vi "Generation word specific.vi"(0 "Template Path":path, 1 "paper size (letter)":i32(ring)=2 items=["wdPaper10x14", "wdPaper11x17", "wdPaperLetter", "wdPaperLetterSmall", "wdPaperLegal", "wdPaperExecutive", "wdPaperA3", "wdPaperA4", "wdPaperA4Small", "wdPaperA5", "wdPaperB4", "wdPaperB5", "wdPaperCSheet", "wdPaperDSheet", "wdPaperESheet", "wdPaperFanfoldLegalGerman", "wdPaperFanfoldStdGerman", "wdPaperFanfoldUS", "wdPaperFolio", "wdPaperLedger", "wdPaperNote", "wdPaperQuarto", "wdPaperStatement", "wdPaperTabloid", "wdPaperEnvelope9", "wdPaperEnvelope10", "wdPaperEnvelope11", "wdPaperEnvelope12", "wdPaperEnvelope14", "wdPaperEnvelopeB4", "wdPaperEnvelopeB5", "wdPaperEnvelopeB6", "wdPaperEnvelopeC3", "wdPaperEnvelopeC4", "wdPaperEnvelopeC5", "wdPaperEnvelopeC6", "wdPaperEnvelopeC65", "wdPaperEnvelopeDL", "wdPaperEnvelopeItaly", "wdPaperEnvelopeMonarch", "wdPaperEnvelopePersonal", "wdPaperCustom"], 2 "Data Set Name":string, 3 "column headers":string[](array[string]), 4 "Table Data":string[][](array[string]), 5 "error in (no error)":errorcluster) -> (14 "Report Saved Path":path, 19 "error out":errorcluster)   [LabVIEW 2020]
uses:
  <vilib>/Utility/NIReport.llb/Report Type.ctl
  <vilib>/addons/_office/_exclsub.llb/font.ctl
  <vilib>/Utility/NIReport.llb/Append Text Table to Report (wrap).vi
  <vilib>/addons/_office/word.llb/Word Edit Cell ([str]).vi
  <vilib>/Utility/NIReport.llb/NI_report.lvclass
  <vilib>/Utility/NIReport.llb/NI_ReportGenerationCore.lvlib
  <vilib>/Utility/NIReport.llb/Word/NI_Word.lvclass
  <vilib>/addons/_office/NI_ReportGenerationToolkit.lvlib
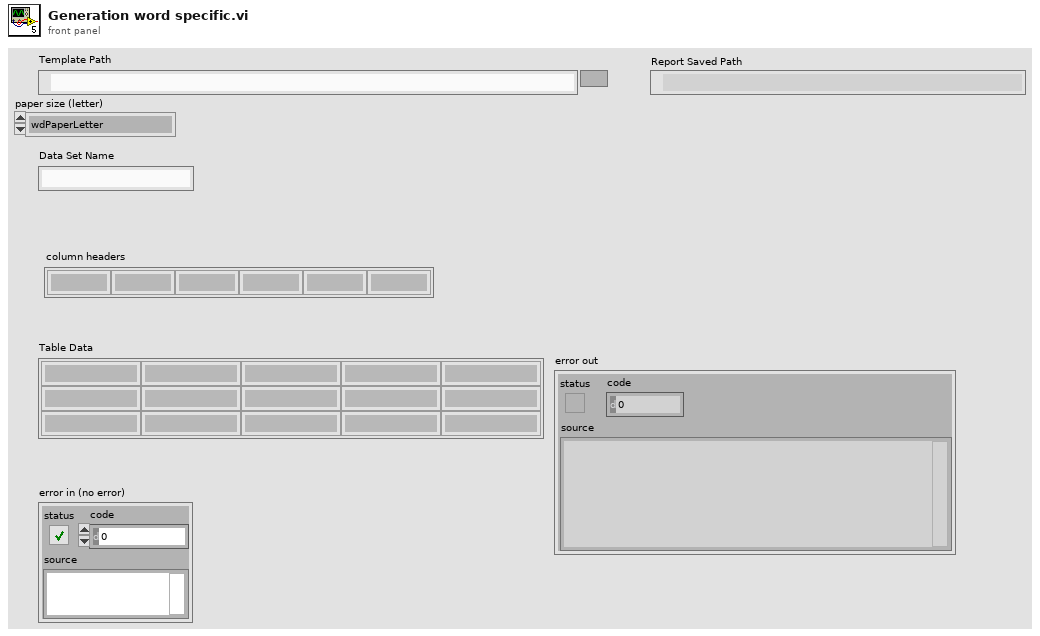
[diagram p1: front panel]
types:
  T1 = typedef "NI_ReportGenerationToolkit.lvlib/font.ctl" = cluster{"font name":string, "font size":dbl, "bold":u16, "italic":u16, "underline":u16, "strike through":u16, "font color":u32}
  T2 = typedef "NI_ReportGenerationCore.lvlib/Report Type.ctl" = enum16{"HTML", "Word", "Excel"}
  T3 = enum16{"maximized", "minimized", "normal", "no change"}
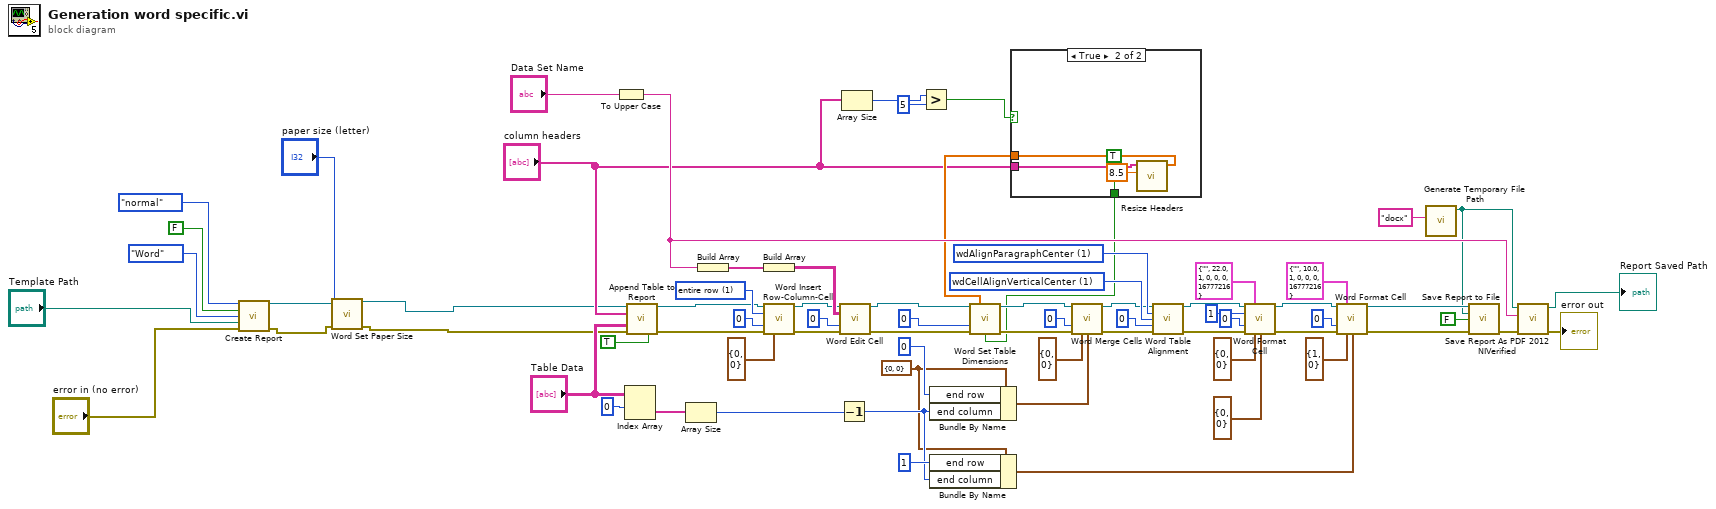
[diagram p0: block diagram]
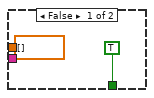
[diagram p2: hidden frame]
diagram:
  w54 = u16 1 items=["shift cells right", "entire row", "entire column"] ("mode (entire column)")
  w24 = cluster{"end row":i32, "end column":i32} {"end row"=0, "end column"=0} ("end")
  w64 = 1 items=["wdCellAlignVerticalTop"=0, "wdCellAlignVerticalCenter"=1, "wdCellAlignVerticalBottom"=3] ("vertical alignment (top)")
  w65 = 1 items=["wdAlignParagraphLeft"=0, "wdAlignParagraphCenter"=1, "wdAlignParagraphRight"=2, "wdAlignParagraphJustify"=3, "wdAlignParagraphDistribute"=4, "wdAlignParagraphJustifyMed"=5, "wdAlignParagraphJustifyHi"=7, "wdAlignParagraphJustifyLow"=8] ("horizontal alignment (left)")
  n1 = call <vilib>:"Create Report.vi"("window state (normal)"=T3."normal", "display alerts? (F)"=FALSE, "report type"=Report_Type."Word", "template (empty)"="Template Path", "error in (no error)"="error in (no error)") -> ("report out"=w6:refnum<class "NI_report.lvclass">, "error out"=w3:errorcluster)  [unwired: 9 in]
  n2 = call <vilib>:"Word Set Paper Size.vi"("report in"=w6, "paper size (letter)"="paper size (letter)", "error in (no error)"=w3) -> ("report out"=w5:refnum<class "NI_report.lvclass">, "error out"=w4:errorcluster)  [unwired: 11 in]
  n3 = To Upper Case(1:"Data Set Name") -> (0:w17:string)
  n4 = Index Array(array="Table Data", index (row)=0) -> (element=w56:string[])  [unwired: 1 in]
  n5 = call-poly <vilib>:"Append Table to Report.vi"("report in"=w5, "column headers"="column headers", "text data"="Table Data", "error in (no error)"=w4, "show grid lines (YES)"=TRUE) -> ("report out"=w8:refnum<class "NI_report.lvclass">, "error out"=w55:errorcluster)  [unwired: 7 in, 2 out]
  n6 = Array Size(array=w56) -> (size(s)=w48:i32)
  n7 = Build Array(w17) -> (w50:string[])
  n8 = Build Array(w50) -> (w49:string[][])
  n9 = call <vilib>:"Word Insert Row-Column-Cell.vi"("report in"=w8, "mode (entire column)"=w54, "table index (-1)"=i16 0, "error in (no error)"=w55, "start (0, 0)"=cluster{"row":i32, "column":i32} {"row"=0, "column"=0}) -> ("report out"=w9:refnum<class "NI_report.lvclass">, "error out"=w51:errorcluster)  [unwired: 9 in]
  n10 = Decrement(x=w48) -> (x-1=w26:i32)
  n11 = call-poly <vilib>:"Word Edit Cell.vi"("report in"=w9, "value"=w49, "table index (-1)"=i16 0, "error in (no error)"=w51) -> ("report out"=w47:refnum<class "NI_report.lvclass">, "error out"=w46:errorcluster)  [unwired: 10 in]
  n12 = Array Size(array="column headers") -> (size(s)=w13:i32)
  n13 = Greater?(x=w13, y=5) -> (0:w11:bool)
  n14 = Bundle By Name(cluster=w24, "end row"=0, "end column"=w26) -> (w59:cluster{"end row":i32, "end column":i32})
  n15 = Bundle By Name(cluster=w24, "end row"=1, "end column"=w26) -> (w25:cluster{"end row":i32, "end column":i32})
  n16 = case shown="True" w11 {
    tunnel: [dbl[] [] ("Resized") w76] -> w15
    tunnel: "column headers" -> [_ w75]
    tunnel: [TRUE ("fit to page width? (F)") TRUE ("fit to page width? (F)")] -> w10
    frame False {
    }
    frame True {
      n17 = call "Resize Headers.vi"("Total Size"=8.5, "Column Headers"=w75) -> ("Resized"=w76:dbl[])  [unwired: 7 in, 2 out]
    }
  }
  n18 = call <vilib>:"Word Set Table Dimensions.vi"("report in"=w47, "table column widths"=w15, "table index (-1)"=i16 0, "error in (no error)"=w46, "fit to page width? (F)"=w10) -> ("report out"=w45:refnum<class "NI_report.lvclass">, "error out"=w44:errorcluster)  [unwired: 9 in]
  n19 = call <vilib>:"Word Merge Cells.vi"("report in"=w45, "table index (-1)"=i16 0, "error in (no error)"=w44, "start (0, 0)"=cluster{"start row":i32, "start column":i32} {"start row"=0, "start column"=0}, "end"=w59) -> ("report out"=w43:refnum<class "NI_report.lvclass">, "error out"=w42:errorcluster)  [unwired: 9 in]
  n20 = call <vilib>:"Word Table Alignment.vi"("report in"=w43, "horizontal alignment (left)"=w65, "vertical alignment (top)"=w64, "table index (-1)"=i16 0, "error in (no error)"=w42) -> ("report out"=w41:refnum<class "NI_report.lvclass">, "error out"=w40:errorcluster)  [unwired: 9 in]
  n21 = call <vilib>:"Word Format Cell.vi"("report in"=w41, "font"=T1 {"font name"="", "font size"=22.0, "bold"=1, "italic"=0, "underline"=0, "strike through"=0, "font color"=16777216}, "autoformat (-1: none)"=1, "table index (-1)"=i16 0, "error in (no error)"=w40, "start (-1, -1)"=cluster{"start row":i32, "start column":i32} {"start row"=0, "start column"=0}, "end (-1, -1)"=cluster{"end row":i32, "end column":i32} {"end row"=0, "end column"=0}) -> ("report out"=w35:refnum<class "NI_report.lvclass">, "error out"=w34:errorcluster)  [unwired: 7 in]
  n22 = call <vilib>:"Word Format Cell.vi"("report in"=w35, "font"=T1 {"font name"="", "font size"=10.0, "bold"=1, "italic"=0, "underline"=0, "strike through"=0, "font color"=16777216}, "table index (-1)"=i16 0, "error in (no error)"=w34, "start (-1, -1)"=cluster{"start row":i32, "start column":i32} {"start row"=1, "start column"=0}, "end (-1, -1)"=w25) -> ("report out"=w33:refnum<class "NI_report.lvclass">, "error out"=w32:errorcluster)  [unwired: 8 in]
  n23 = call <vilib>:"Generate Temporary File Path.vi"("Temporary File Extension (tmp)"="docx") -> ("Unique Temporary File Path"=w1:path)  [unwired: 9 in, 1 out]
  n24 = call-dynamic "Save Report to File.vi"("report in"=w33, "report file path"=w1, "prompt to replace? (F)"=FALSE, "error in (no error)"=w32) -> ("error out"=w18:errorcluster)  [unwired: 10 in, 1 out]
  n25 = call "Save Report As PDF 2012 NIVerified.vi"("error in (no error)"=w18, "Data Set Name"=w17, "Report file path"=w1) -> ("error out"=→"error out":errorcluster, "Report Saved Path"=→"Report Saved Path":path)  [unwired: 7 in]
